vi "optionsAcq_channel_select.vi"(8 "error in (no error)":errorcluster, 9 "channelType_spectrum":T1, 10 "channel DUT (index)":i32, 11 "Thorlabs_OSA200_64 in":refnum<class "OSA200.lvclass">) -> (0 "error out":errorcluster, 2 "channel DUT out":i32, 3 "Thorlabs_OSA200_64 out":refnum<class "OSA200.lvclass">)   [LabVIEW 2010, in "OSA200.lvclass"]
uses:
  OSA200.lvclass
  _misc/Thorlabs_FTS_misc.llb/channelType_spectrum.ctl
  OSA.lvclass
  OSA20X_misc.lvlib
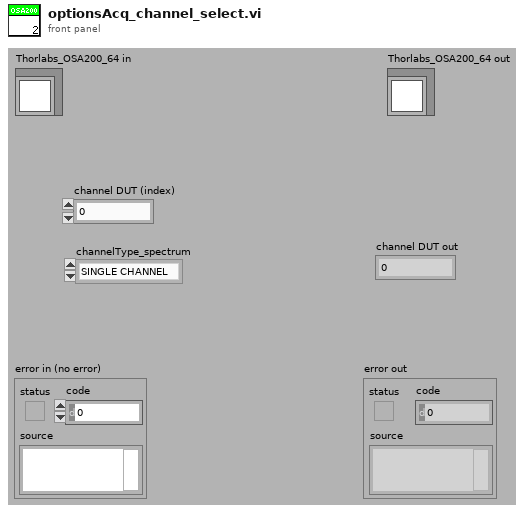
[diagram p1: front panel]
types:
  T1 = typedef "OSA20X_misc.lvlib/channelType_spectrum.ctl" = enum16{"SINGLE CHANNEL", "STICHED"}
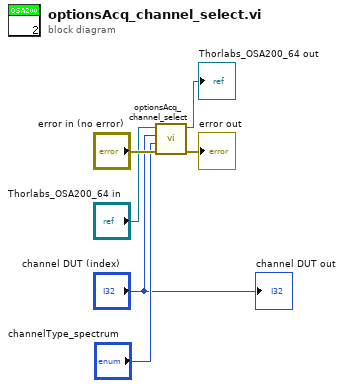
[diagram p0: block diagram]
diagram:
  n1 = call-parent "optionsAcq_channel_select.vi"("error in (no error)"="error in (no error)", "channelType_spectrum"="channelType_spectrum", "channel DUT (index)"="channel DUT (index)", "Thorlabs_OSA_64 in"="Thorlabs_OSA200_64 in") -> ("error out"=→"error out":errorcluster, "Thorlabs_OSA_64 out"=→"Thorlabs_OSA200_64 out":refnum<class "OSA200.lvclass">)  [unwired: 5 in, 1 out]
  "channel DUT out" <- "channel DUT (index)"
